vi "Set Power.vi"(8 "error in (no error)":errorcluster, 10 "Power":i32 min=0 max=5 step=1, 11 "Julabo FP-50 Settings":T1) -> (0 "error out":errorcluster, 1 "Connection Error":bool, 3 "Julabo FP-50 Settings":T1)   [LabVIEW 2021]
uses:
  Third Party Drivers/Julabo Type 1/JULABO DeviceDriver/JULABO DeviceDriver.lvlib
  HotCoil Settings.ctl
  HotCoil.lvlib
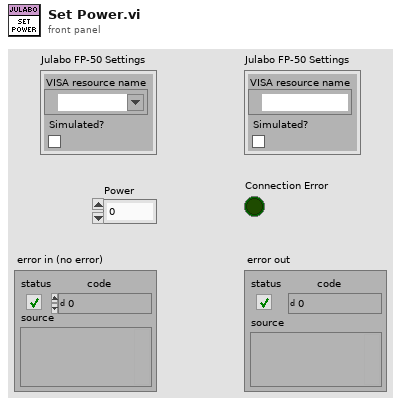
[diagram p1: front panel]
types:
  T1 = typedef "HotCoil.lvlib/HotCoil Settings.ctl" = cluster{"VISA resource name":refnum<visa-resource-name>, "Simulated?":bool}
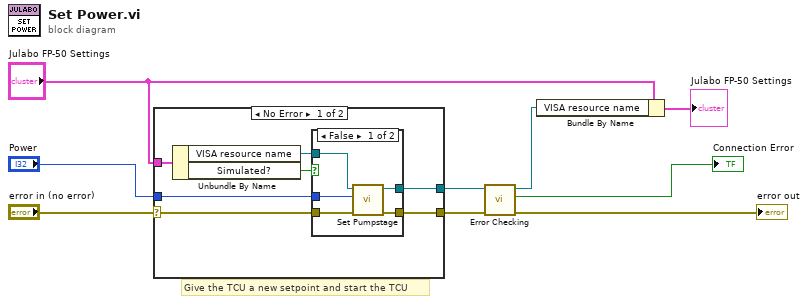
[diagram p0: block diagram]
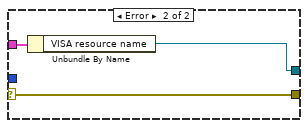
[diagram p3: hidden frame]
diagram:
  # "Give the TCU a new setpoint and start the TCU"
  n1 = case shown="No Error" "error in (no error)" {
    selector: "error in (no error)" -> [w16 w26]
    tunnel: "Julabo FP-50 Settings" -> [w12 w25]
    tunnel: [w15 w26] -> w7
    tunnel: [w14 w24] -> w8
    tunnel: "Power" -> [w10 _]
    frame No Error {
      n2 = Unbundle By Name(w12) -> ("VISA resource name"=w11:refnum<visa-resource-name>, "Simulated?"=w13:bool)
      n3 = case shown="False" w13 {
        tunnel: w16 -> [w18 w23]
        tunnel: [w17 w23] -> w15
        tunnel: [w20 w22] -> w14
        tunnel: w11 -> [w21 w22]
        tunnel: w10 -> [w19 _]
        frame False {
          n4 = call "Set Pumpstage.vi"("error in (no error)"=w18, "Pumpstage (1: default)"=w19, "VISA resource name"=w21) -> ("error out"=w17:errorcluster, "VISA resource name out"=w20:refnum<visa-resource-name>)  [unwired: 7 in]
        }
        frame True {
        }
      }
    }
    frame Error {
      n5 = Unbundle By Name(w25) -> ("VISA resource name"=w24:refnum<visa-resource-name>)
    }
  }
  n6 = call "Error Checking.vi"("error in (no error)"=w7, "VISA resource name"=w8) -> ("error out"=→"error out":errorcluster, "Connection Error"=→"Connection Error":bool, "VISA resource name"=w5:refnum<visa-resource-name>)  [unwired: 7 in]
  n7 = Bundle By Name(cluster="Julabo FP-50 Settings", "VISA resource name"=w5) -> (→"Julabo FP-50 Settings":T1)
